vi "Limit Switch Init.vi"(1 "error in":errorcluster) -> (0 "error out":errorcluster)   [LabVIEW 2014]
uses:
  <vilib>/Rock Robotics/SystemInterfaces/DIO/FPGA_DIOChannel.ctl
  <vilib>/Rock Robotics/SystemInterfaces/Typedef/FPGA_TypedefDigitalModule.ctl
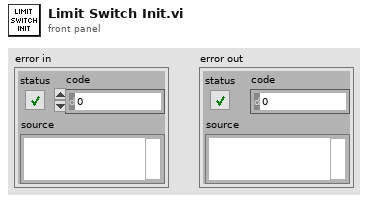
[diagram p1: front panel]
types:
  T1 = typedef "FPGA_DIOChannel.ctl" = enum8{"DIO 0", "DIO 1", "DIO 2", "DIO 3", "DIO 4", "DIO 5", "DIO 6", "DIO 7", "DIO 8", "DIO 9", "DIO MXP 0", "DIO MXP 1", "DIO MXP 2", "DIO MXP 3", "DIO MXP 4", "DIO MXP 5", "DIO MXP 6", "DIO MXP 7", "DIO MXP 8", "DIO MXP 9", "DIO MXP 10", "DIO MXP 11", "DIO MXP 12", "DIO MXP 13", "DIO MXP 14", "DIO MXP 15", "Invalid"}
  T2 = typedef "FPGA_TypedefDigitalModule.ctl" = enum16{"Controller 1"}
  T3 = typedef "WPI_DigitalInputDevRef.ctl" = cluster{"DevStatus":errorcluster, "DIO Channel":T1, "Controller":T2}
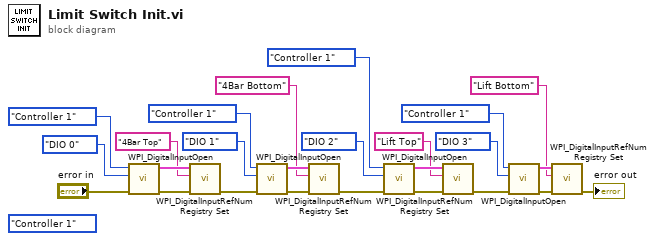
[diagram p0: block diagram]
diagram:
  (unwired) FPGA_TypedefDigitalModule."Controller 1" ("Controller")
  n1 = call <vilib>:"WPI_DigitalInputOpen.vi"("error in (no error)"="error in", "DIO Channel"=FPGA_DIOChannel."DIO 0", "Controller"=FPGA_TypedefDigitalModule."Controller 1") -> ("error out"=w20:errorcluster, "DigitalInputDevRef"=w22:T3)  [unwired: 7 in]
  n2 = call <vilib>:"WPI_DigitalInputRefNum Registry Set.vi"("error in (no error)"=w20, "refnum name"="4Bar Top", "DigitalInputDevRef"=w22) -> ("error out"=w11:errorcluster)  [unwired: 7 in, 1 out]
  n3 = call <vilib>:"WPI_DigitalInputOpen.vi"("error in (no error)"=w11, "DIO Channel"=FPGA_DIOChannel."DIO 1", "Controller"=FPGA_TypedefDigitalModule."Controller 1") -> ("error out"=w18:errorcluster, "DigitalInputDevRef"=w19:T3)  [unwired: 7 in]
  n4 = call <vilib>:"WPI_DigitalInputRefNum Registry Set.vi"("error in (no error)"=w18, "refnum name"="4Bar Bottom", "DigitalInputDevRef"=w19) -> ("error out"=w9:errorcluster)  [unwired: 7 in, 1 out]
  n5 = call <vilib>:"WPI_DigitalInputOpen.vi"("error in (no error)"=w9, "DIO Channel"=FPGA_DIOChannel."DIO 2", "Controller"=FPGA_TypedefDigitalModule."Controller 1") -> ("error out"=w16:errorcluster, "DigitalInputDevRef"=w17:T3)  [unwired: 7 in]
  n6 = call <vilib>:"WPI_DigitalInputRefNum Registry Set.vi"("error in (no error)"=w16, "refnum name"="Lift Top", "DigitalInputDevRef"=w17) -> ("error out"=w3:errorcluster)  [unwired: 7 in, 1 out]
  n7 = call <vilib>:"WPI_DigitalInputOpen.vi"("error in (no error)"=w3, "DIO Channel"=FPGA_DIOChannel."DIO 3", "Controller"=FPGA_TypedefDigitalModule."Controller 1") -> ("error out"=w14:errorcluster, "DigitalInputDevRef"=w15:T3)  [unwired: 7 in]
  n8 = call <vilib>:"WPI_DigitalInputRefNum Registry Set.vi"("error in (no error)"=w14, "refnum name"="Lift Bottom", "DigitalInputDevRef"=w15) -> ("error out"=→"error out":errorcluster)  [unwired: 7 in, 1 out]
